vi "Attention Message.vi"(1 "Error In":errorcluster) -> (0 "Error Out":errorcluster)   [LabVIEW 2013]
panel:
  in  "OK Button":bool
  # "Please check settings!"
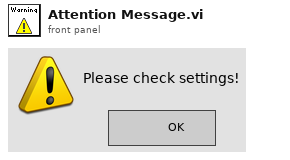
[diagram p1: front panel]
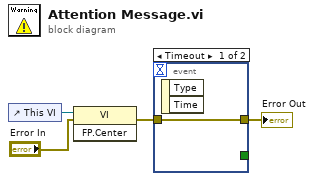
[diagram p0: block diagram]
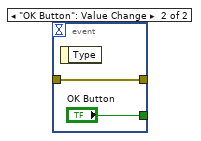
[diagram p2: hidden frame]
diagram:
  n1 = control-ref of="This VI"() -> (w4:refnum<vi>)
  n2 = invoke class="VI" method="FP.Center"(reference=w4, error in="Error In") -> (error out=w3:errorcluster)  [unwired: 1 in, 2 out]
  n3 = event shown="[0] Timeout" {
    selector: _ -> [_ _]
    dyn-events: _ -> [_ _]
    timeout: _ -> [_ _]
    tunnel: [_ "OK Button"] -> _
    tunnel: w3 -> [w5 w6]
    tunnel: [w5 w6] -> w2
    event Timeout {
      n4 = event-data() -> ()  [unwired: 1 in, 2 out]
    }
    event "OK Button": Value Change {
      n5 = event-data() -> ()  [unwired: 1 in, 1 out]
    }
  }
  "Error Out" <- w2
